vi "globalMessage.vi"() -> ()   [LabVIEW 2018]
panel:
  out "心跳返回值":i32
  out "近场相机链接":bool
  out "是否完成本次测量？":bool
  out "首次设置任务？":bool=TRUE
  out "实时消息1":T1
  in  "当前运行信息":string
  # "功率计"
  # "能量计"
  # "时间波形"
  # "光谱"
  # "偏振"
  # "近远场"
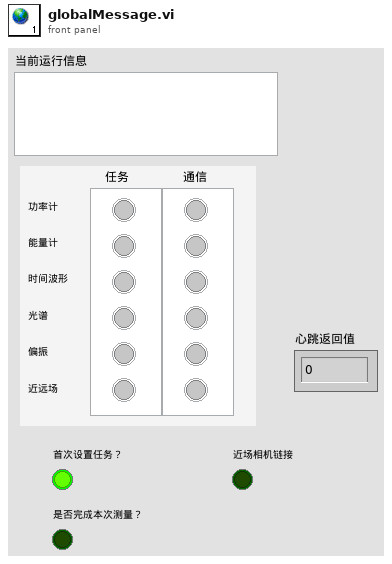
[diagram p1: front panel]
types:
  T1 = cluster{"任务":cluster{"功率任务":bool, "能量任务":bool, "时间波形任务":bool, "光谱任务":bool, "偏振任务":bool, "近远场任务":bool}, "通信":cluster{"功率通信":bool, "能量通信":bool, "时间波形通信":bool, "光谱通信":bool, "偏振通信":bool, "近远场通信":bool}}
diagram:
